vi "Write System Name.vi"(8 "error in (no error)":errorcluster, 10 "System Name":string, 11 "crio configuration in":refnum<class "cRIO configuration.lvclass">) -> (0 "error out":errorcluster, 3 "crio configuration out":refnum<class "cRIO configuration.lvclass">)   [LabVIEW 2013, in "crio configuration.lvclass"]
uses:
  cRIO configuration.lvclass
  Configuration Framework/serializable configuration/NISE_CEF_serializable configuration.lvclass
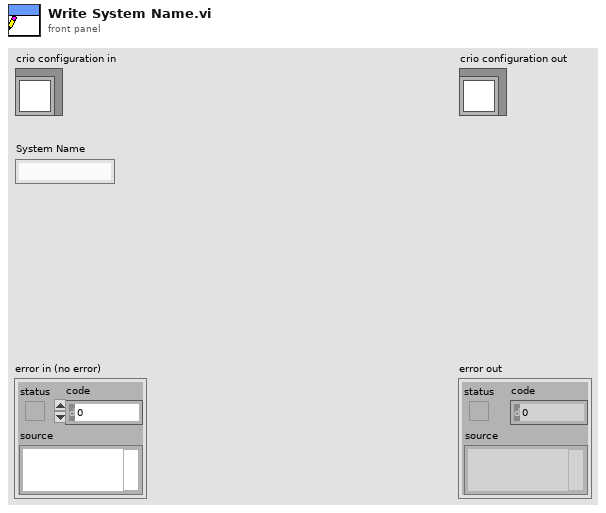
[diagram p1: front panel]
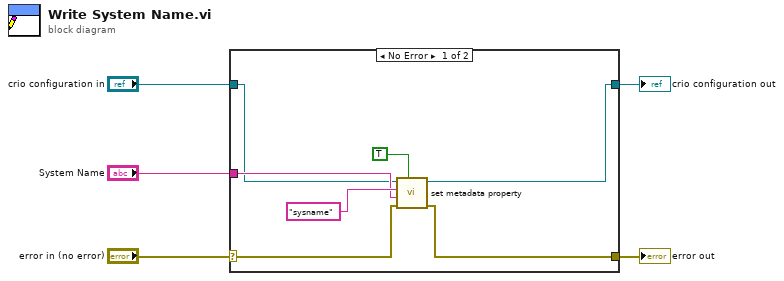
[diagram p0: block diagram]
diagram:
  n1 = case shown="No Error" "error in (no error)" {
    selector: "error in (no error)" -> [w12 w13]
    tunnel: [w6 w13] -> w4
    tunnel: [w7 w14] -> w2
    tunnel: "crio configuration in" -> [w8 w14]
    tunnel: "System Name" -> [w10 _]
    frame No Error {
      n2 = call "set metadata property.vi"("overwrite?"=TRUE, "error in"=w12, "value"=w10, "key"="sysname", "configuration in"=w8) -> ("error out"=w6:errorcluster, "configuration out"=w7:refnum<class "cRIO configuration.lvclass">)  [unwired: 5 in]
    }
    frame Error {
    }
  }
  "error out" <- w4
  "crio configuration out" <- w2
